vi "VoltageTest.vi"() -> ()   [LabVIEW 2017]
uses:
  <vilib>/Platform/TimedLoop/XDataNode/timing_clust.ctl
  <vilib>/Platform/TimedLoop/XDataNode/nitl_modes.ctl
  <vilib>/Platform/TimedLoop/XDataNode/wakeup.ctl
  <vilib>/FPGAPlugInAG/cRIO-9065/niLvFpga_Open_cRIO-9065.vi
  <vilib>/rvi/interface/common/dynamic/niFpgaDynamicAddResources.vi
  <vilib>/Utility/error.llb/Error Cluster From Error Code.vi
  <vilib>/rvi/errors/niLvFpgaAdjustHostInterfaceError.vi
  <vilib>/FPGAPlugInAG/Dynamic/niLvFpga_Run_Dynamic.vi
  <vilib>/FPGAPlugInAG/Dynamic/niLvFpga_Abort_Dynamic.vi
  <vilib>/platform/TimedLoop/XDataNode/XDataNode.xnode
  <vilib>/rvi/interface/nirviOpenFPGA/nirviOpenFPGA.xnode
  FPGA Bitfiles/fpgaproject_FPGATarget_fpgamain2_a5SRlSt3u8Q.lvbitx
  Fpga.vi
  <vilib>/rvi/interface/nirviMethod/nirviMethod.xnode
  <vilib>/rvi/interface/nirviReadWriteControl/nirviReadWriteControl.xnode
  NiFpgaLv.dll
  <vilib>/rvi/interface/Simulation/niFpgaSimulationCallBeginRW.vi
  <vilib>/Platform/TimedLoop/XDataNode/XDNodeRunTimeDep.lvlib
  <vilib>/FPGAPlugInAG/Dynamic/niLvFpga_StartFifo_Dynamic.vi
  <vilib>/rvi/errors/niLvFpgaMergeErrorWithErrorCode.vi
panel:
  in  "Numeric Control":dbl
  out "Velocity":cluster{dbl[], dbl[]}(graph)
  out "Voltage Position":cluster{dbl[], dbl[]}(graph)
  in  "Save Data Name":string
  in  "Period":i64=1
  in  "Voltage In":fxp<+/-,64,32>
  in  "stop":bool
  out "time loop error":errorcluster
  out "速率":dbl
  in  "Position Reset":bool
  out "Encoder Position":dbl format="%#_8g"
  out "Voltage Out":fxp<+/-,20,5>
  out "Real Period":u32
  out "沖壓":bool
  out "結束了":bool
  out "shutdown error":errorcluster
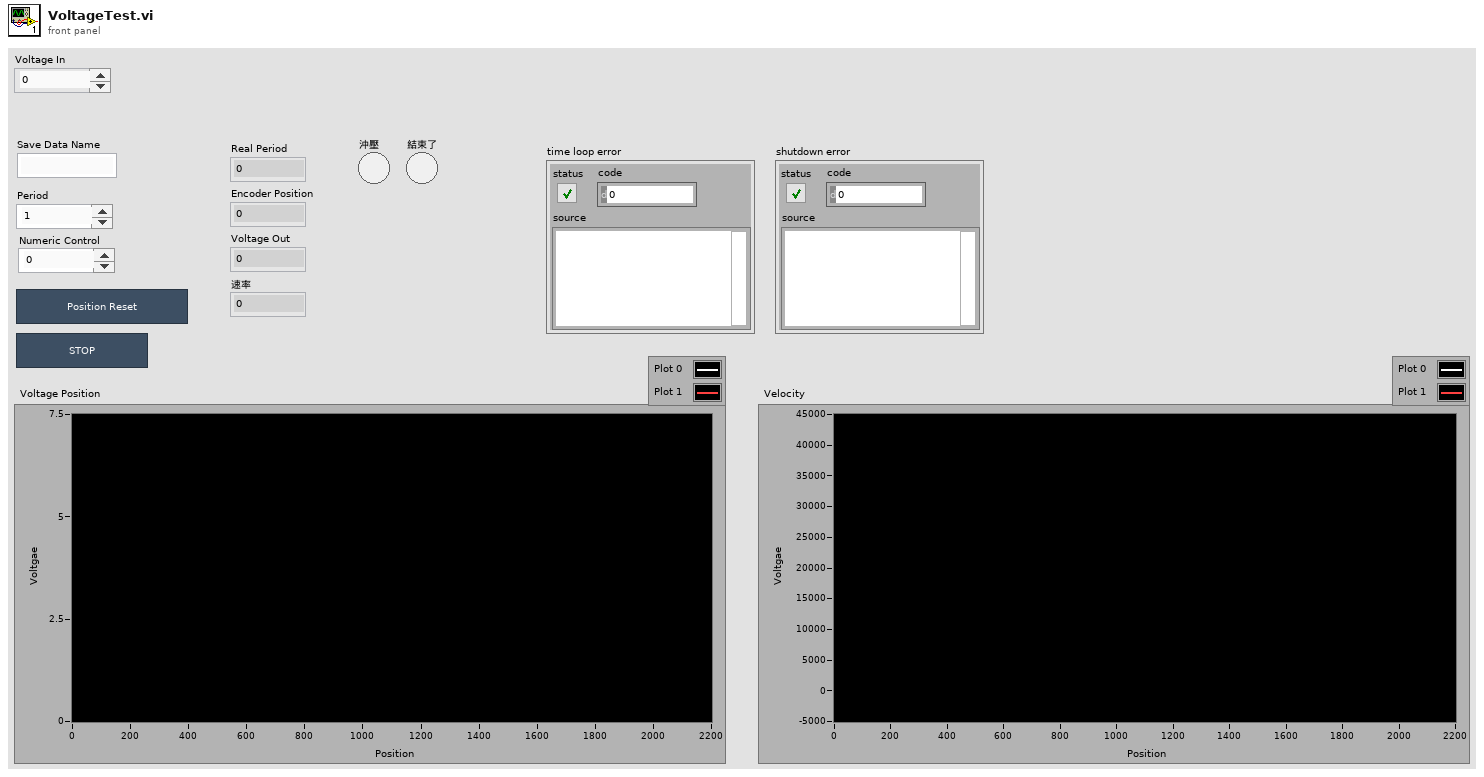
[diagram p1: front panel]
types:
  T1 = enum16{"open", "replace", "create", "open or create", "replace or create", "replace or create with confirmation"}
  T2 = typedef "XDNodeRunTimeDep.lvlib/timing_clust.ctl" = cluster{"Expected End [f-1]":u64, "Actual End [f-1]":u64, "Finished Late? [f-1]":bool, "Expected End [i-1]":u64, "Actual End [i-1]":u64, "Finished Late? [i-1]":bool, "Expected Start [i]":u64, "Actual Start [i]":u64, "Expected Start [f]":u64, "Actual Start [f]":u64, "Source Name":string, "Structure Name":string, "Period":i64, "Deadline":i64, "Offset":i64, "Start":i64, "Priority":i32, "Timeout":i32, "Mode":T3, "Wakeup Reason":T4, "Error":errorcluster, "Source Type":string, "Secondary Source Type":string, "Global End Time":u64, "Global Start Time":u64, "Frame Duration":u64, "Iteration Duration":u64, "Assigned CPU":i32, "I/O Scan Engine Mode":u32}
  T3 = typedef "XDNodeRunTimeDep.lvlib/nitl_modes.ctl" = enum32{"No Change", "Process missed periods, maintain original phase", "Discard missed periods, maintain original phase", "Process missed periods, ignore original phase", "Discard missed periods, ignore original phase"}
  T4 = typedef "XDNodeRunTimeDep.lvlib/wakeup.ctl" = enum32{"Normal", "Aborted", "Asynchronous wakeup", "Timing source error", "Timed loop error", "Timeout"}
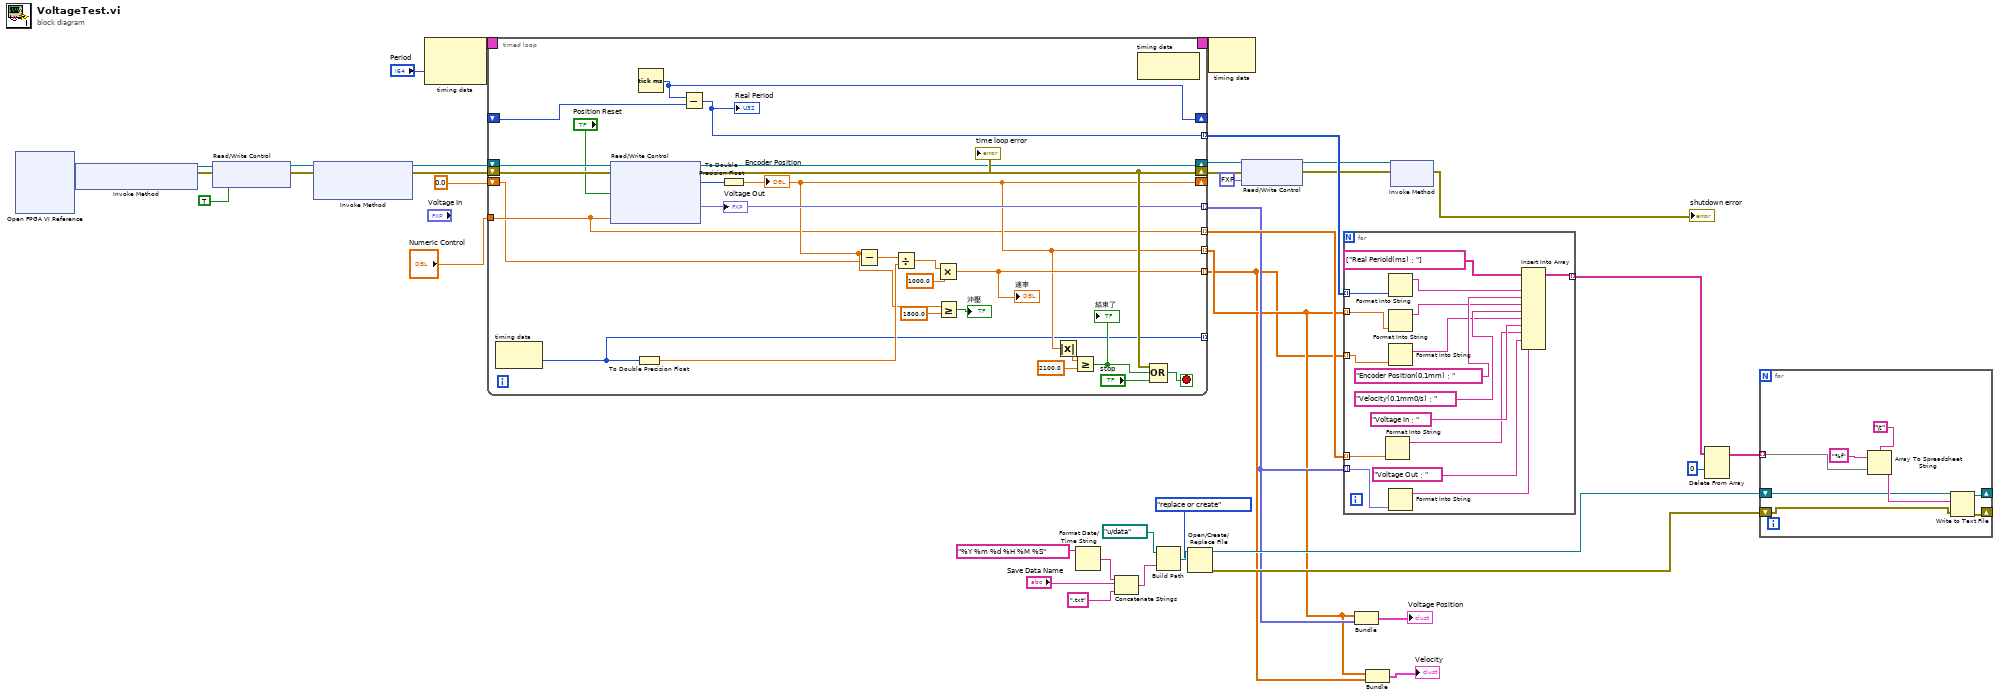
[diagram p0: block diagram]
diagram:
  n1 = xnode "Open FPGA VI Reference"() -> ("FPGA VI Reference Out"=w32:refnum<k20>, "error out"=w31:errorcluster)  [unwired: 2 in]
  n2 = xnode "Invoke Method"("FPGA VI Reference In"=w32, "error in"=w31) -> ("FPGA VI Reference Out"=w30:refnum<k20>, "error out"=w29:errorcluster)
  n3 = xnode "Read/Write Control"("FPGA VI Reference In"=w30, "error in"=w29, "Position Reset"=TRUE) -> ("FPGA VI Reference Out"=w28:refnum<k20>, "error out"=w27:errorcluster)
  n4 = xnode "Invoke Method"("FPGA VI Reference In"=w28, "error in"=w27) -> ("FPGA VI Reference Out"=w38:refnum<k20>, "error out"=w37:errorcluster)  [unwired: 1 in]
  n5 = node-c288("Period") -> (w40:T2)  [unwired: 1 in]
  n6 = timed-loop {
    shift-right: [w64] -> w10
    shift-left: w38 -> [w63]
    shift-right: [w58] -> w9
    shift-left: w37 -> [w65]
    timing: w40 -> [_]
    timing-out: [_] -> w39
    shift-right: [w49] -> _
    shift-left: 0.0 -> [w41]
    tunnel: [w49] -> w3 mode=indexing
    tunnel: [w55] -> w2 mode=indexing
    tunnel: [w53] -> w13 mode=indexing
    tunnel: [w45] -> _ mode=indexing
    shift-right: [w51] -> _
    shift-left: _ -> [w52]
    tunnel: [w50] -> w34 mode=indexing
    tunnel: "Numeric Control" -> [w43]
    tunnel: [w43] -> w33 mode=indexing
    stop <- w60 stop-if-true
    n7 = node-c288() -> (w45:i64)  [unwired: 1 in]
    n8 = xnode "Read/Write Control"("FPGA VI Reference In"=w63, "error in"=w65, "Position Reset"="Position Reset", "Vlotage In"=w43) -> ("FPGA VI Reference Out"=w64:refnum<k20>, "error out"=w58:errorcluster, "Position (Counts)"=w44:i32, "Voltage Out"=w53:fxp<+/-,20,5>)
    "Voltage Out" <- w53
    n9 = To Double Precision Float(number=w45) -> (double precision float=w57:dbl)
    n10 = Tick Count (ms)() -> (millisecond timer value=w51:u32)
    n11 = Subtract(x=w51, y=w52) -> (x-y=w50:u32)
    "Real Period" <- w50
    n12 = To Double Precision Float(number=w44) -> (double precision float=w49:dbl)
    "Encoder Position" <- w49
    n13 = Subtract(x=w49, y=w41) -> (x-y=w66:dbl)
    n14 = Divide(x=w66, y=w57) -> (x/y=w56:dbl)
    n15 = Multiply(x=w56, y=1000.0) -> (x*y=w55:dbl)
    "速率" <- w55
    n16 = Greater Or Equal?(x=w49, y=1800.0) -> (x >= y?=→"沖壓":bool)
    n17 = Absolute Value(x=w49) -> (abs(x)=w54:dbl)
    n18 = Greater Or Equal?(x=w54, y=2100.0) -> (x >= y?=w46:bool)
    "結束了" <- w46
    n19 = node-c288() -> ()  [unwired: 1 in, 1 out]
    n20 = Compound Arithmetic op=OR(w58, w46, "stop") -> (w60:bool)
    "time loop error" <- w65
  }
  n21 = Format Date/Time String(time format string (%c)="%Y %m %d %H %M %S") -> (date/time string=w25:string)  [unwired: 2 in]
  n22 = Concatenate Strings(w25, "Save Data Name", ".txt" ("element")) -> (w24:string)
  n23 = Build Path(base path=path "u:/data", name or relative path=w24) -> (appended path=w26:path)
  n24 = Open/Create/Replace File(file path (use dialog)=w26, operation (0:open)=T1."replace or create") -> (refnum out=w16:refnum<file>, error out=w15:errorcluster)  [unwired: 4 in, 1 out]
  n25 = node-c288(w39) -> ()  [unwired: 1 out]
  n26 = xnode "Read/Write Control"("FPGA VI Reference In"=w10, "error in"=w9, "Vlotage In"=fxp<+/-,20,5> 0.0) -> ("FPGA VI Reference Out"=w8:refnum<k20>, "error out"=w7:errorcluster)
  n27 = for {
    tunnel: [w83] -> w19 mode=indexing
    tunnel: w3 -> [w80] mode=indexing
    tunnel: w2 -> [w82] mode=indexing
    tunnel: w13 -> [w76] mode=indexing
    tunnel: w34 -> [w75] mode=indexing
    tunnel: w33 -> [w70] mode=indexing
    n28 = Format Into String(w70) -> (resulting string=w73:string)  [unwired: 3 in, 1 out]
    n29 = Format Into String(w75) -> (resulting string=w78:string)  [unwired: 3 in, 1 out]
    n30 = Format Into String(w80) -> (resulting string=w79:string)  [unwired: 3 in, 1 out]
    n31 = Format Into String(w82) -> (resulting string=w81:string)  [unwired: 3 in, 1 out]
    n32 = Format Into String(w76) -> (resulting string=w71:string)  [unwired: 3 in, 1 out]
    n33 = Insert Into Array(array=string[] ["Real Periold(ms)："], new element #1=w78, new element #2="Encoder Position(0.1mm)：", new element #3=w79, new element #4="Velocity(0.1mm0/s)：", new element #5=w81, new element #6="Voltage In：", new element #7=w73, new element #8="Voltage Out：", new element #9=w71) -> (w83:string[])  [unwired: 1 in]
  }
  n34 = Bundle(w3, w13) -> (→"Voltage Position":cluster{dbl[], fxp<+/-,20,5>[]})  [unwired: 1 in]
  n35 = Bundle(w3, w2) -> (→"Velocity":cluster{dbl[], dbl[]})  [unwired: 1 in]
  n36 = xnode "Invoke Method"("FPGA VI Reference In"=w8, "error in"=w7) -> ("error out"=→"shutdown error":errorcluster)  [unwired: 1 out]
  n37 = Delete From Array(array=w19, index (row)=0) -> (array with subset deleted=w17:string[][])  [unwired: 2 in, 1 out]
  n38 = for {
    shift-right: [w87] -> _
    shift-left: w16 -> [w90]
    shift-right: [w88] -> _
    shift-left: w15 -> [w89]
    tunnel: w17 -> [w86] mode=indexing
    n39 = Array To Spreadsheet String(delimiter (Tab)="\t", array=w86, 3:"%f" ("format string")) -> (spreadsheet string=w91:string)
    n40 = Write to Text File(file (use dialog)=w90, text=w91, error in=w89) -> (refnum out=w87:refnum<file>, error out=w88:errorcluster)  [unwired: 1 in, 1 out]
  }
